vi "Parse Key Value Pair.vi"(8 "error in (no error)":errorcluster, 11 "key value pair":string) -> (0 "error out":errorcluster, 3 "KVC":string[](array[string]))   [LabVIEW 2010, in "NI_LVConfig.lvlib"]
uses:
  NI_LVConfig.lvlib
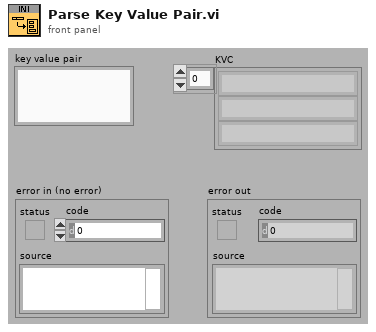
[diagram p1: front panel]
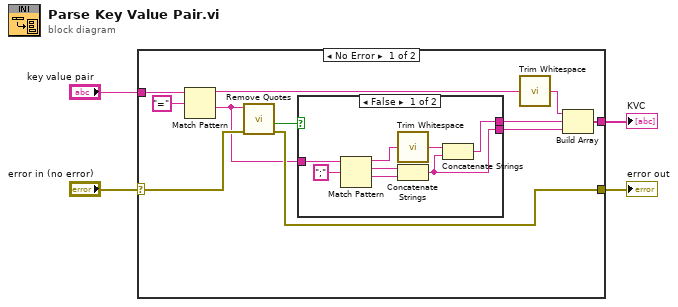
[diagram p0: block diagram]
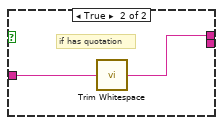
[diagram p2: hidden frame]
diagram:
  n1 = case shown="No Error" "error in (no error)" {
    selector: "error in (no error)" -> [w7 w26]
    tunnel: "key value pair" -> [w14 _]
    tunnel: [w13 _] -> w3
    tunnel: [w6 w26] -> w1
    frame No Error {
      n2 = Match Pattern(string=w14, regular expression="=") -> (before substring=w12:string, after substring=w5:string)  [unwired: 1 in, 2 out]
      n3 = call "Remove Quotes.vi"("error in (no error)"=w7, "string"=w5) -> ("error out"=w6:errorcluster, "in quotes?"=w8:bool)  [unwired: 7 in, 1 out]
      n4 = case shown="False" w8 {
        tunnel: [w16 w25] -> w10
        tunnel: w5 -> [w20 w24]
        tunnel: [w19 _] -> w9
        frame False {
          n5 = Match Pattern(string=w20, regular expression=";") -> (before substring=w17:string, match substring=w22:string, after substring=w23:string)  [unwired: 1 in, 1 out]
          n6 = call "Trim Whitespace.vi"("string"=w17) -> ("trimmed string"=w18:string)  [unwired: 1 in]
          n7 = Concatenate Strings(w22, w23) -> (w19:string)
          n8 = Concatenate Strings(w18, w19) -> (w16:string)
        }
        frame True {
          # "if has quotation"
          n9 = call "Trim Whitespace.vi"("string"=w24) -> ("trimmed string"=w25:string)  [unwired: 1 in]
        }
      }
      n10 = call "Trim Whitespace.vi"("string"=w12) -> ("trimmed string"=w11:string)  [unwired: 1 in]
      n11 = Build Array(w11, w10, w9) -> (w13:string[])
    }
    frame Error {
    }
  }
  "KVC" <- w3
  "error out" <- w1
